vi "CreatePath.vi"(1 "filetype":enum16{".h5", ".txt"}(ring), 2 "FileName":string) -> (0 "File path":path=path "Cluster Attributes.hdf5")   [LabVIEW 2019]
panel:
  out "Task Status":string
  out "error out":errorcluster
  in  "error in (no error)":errorcluster
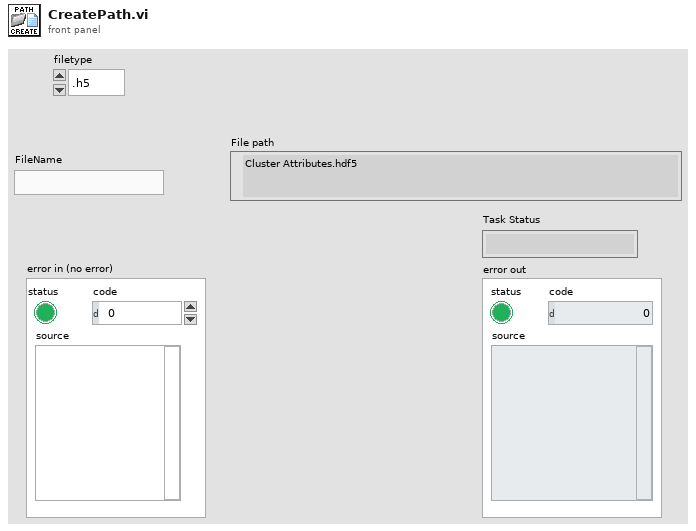
[diagram p1: front panel]
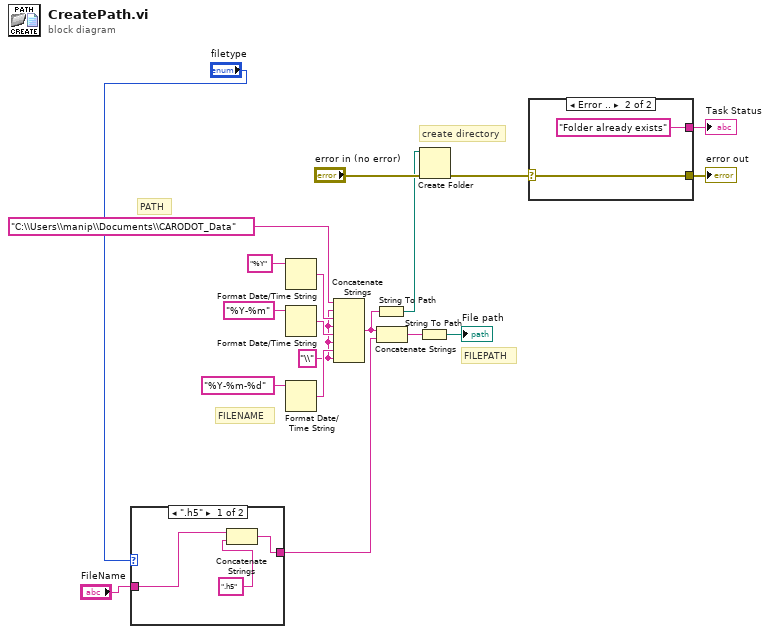
[diagram p0: block diagram]
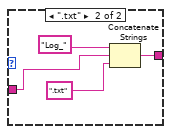
[diagram p2: hidden frame]
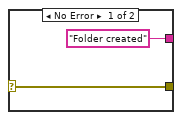
[diagram p3: hidden frame]
diagram:
  w8 = "\\"
  # "FILEPATH"
  # "FILENAME"
  # "PATH"
  # "create directory"
  n1 = case shown="\".h5\"" "filetype" {
    tunnel: [w20 w26] -> w2
    tunnel: "FileName" -> [w22 w25]
    frame ".h5" {
      n2 = Concatenate Strings(w22, ".h5" ("string")) -> (w20:string)
    }
    frame ".txt" {
      n3 = Concatenate Strings("Log_" ("string"), w25, ".txt" ("string")) -> (w26:string)
    }
  }
  n4 = Format Date/Time String(time format string (%c)="%Y") -> (date/time string=w11:string)  [unwired: 2 in]
  n5 = Format Date/Time String(time format string (%c)="%Y-%m") -> (date/time string=w10:string)  [unwired: 2 in]
  n6 = Format Date/Time String(time format string (%c)="%Y-%m-%d") -> (date/time string=w9:string)  [unwired: 2 in]
  n7 = Concatenate Strings("C:\\Users\\manip\\Documents\\CARODOT_Data", w8, w11, w8, w10, w8, w9, w8) -> (w6:string)
  n8 = String To Path(string=w6) -> (path=w4:path)
  n9 = Concatenate Strings(w6, w2) -> (w5:string)
  n10 = String To Path(string=w5) -> (path=→"File path":path)
  n11 = Create Folder(path (use dialog)=w4, error in="error in (no error)") -> (error out=w17:errorcluster)  [unwired: 1 in, 2 out]
  n12 = case shown="Error .." w17 {
    selector: w17 -> [w27 w29]
    tunnel: ["Folder created" "Folder already exists"] -> w16
    tunnel: [w27 w29] -> w18
    frame No Error {
    }
    frame Error {
    }
  }
  "Task Status" <- w16
  "error out" <- w18
